vi "create windowed data.vi"(9 "Window Size":i32, 10 "Window Data":bool, 11 "Array in":dbl[](array[numeric])) -> (3 "Array out":dbl[](array[numeric]))   [LabVIEW 2015]
panel:
  out "Initial Array Size":i32
  out "size(s)":i32
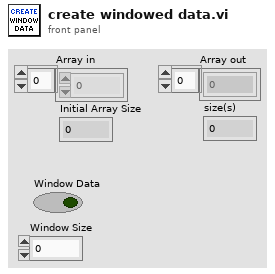
[diagram p1: front panel]
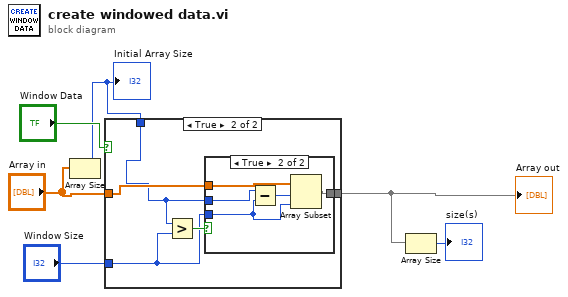
[diagram p0: block diagram]
diagram:
  n1 = Array Size(array="Array in") -> (size(s)=w1:i32)
  "Initial Array Size" <- w1
  n2 = case shown="True" "Window Data" {
    tunnel: "Array in" -> [w7 w10]
    tunnel: [w7 w12] -> w4
    tunnel: "Window Size" -> [_ w9]
    tunnel: w1 -> [_ w8]
    frame False {
    }
    frame True {
      n3 = Greater?(x=w8, y=w9) -> (0:w11:bool)
      n4 = case shown="True" w11 {
        tunnel: w10 -> [w13 w18]
        tunnel: [w13 w17] -> w12
        tunnel: w9 -> [_ w14]
        tunnel: w8 -> [_ w15]
        frame False {
        }
        frame True {
          n5 = Subtract(x=w15, y=w14) -> (x-y=w16:i32)
          n6 = Array Subset(array=w18, index=w16, length=w14) -> (w17:dbl[])
        }
      }
    }
  }
  "Array out" <- w4
  n7 = Array Size(array=w4) -> (size(s)=→"size(s)":i32)
